vi "PH_Sequencer_Watch.PC _PUcharged.vi"(0 "i ref in":refnum<vi>, 2 "Tagname":string, 3 "Tagvalue":i32, 4 "no link":bool, 5 "error in (no error)":errorcluster) -> (14 "i ref out":refnum<vi>, 19 "error out":errorcluster)   [LabVIEW 2014, in "PH_Sequencer_Watch.lvlib"]
doc: "This VI writes the incoming information for measured voltage to the related GUI element and to own attributes."
uses:
  PH_Sequencer_Watch.lvlib
  PH_Basics/PH_PowerUnit_BaseClass/PH_PowerUnit_BaseClass.PP PU Tags.ctl
  PH_Basics/PH_PowerUnit_BaseClass/PH_PowerUnit_BaseClass.lvlib
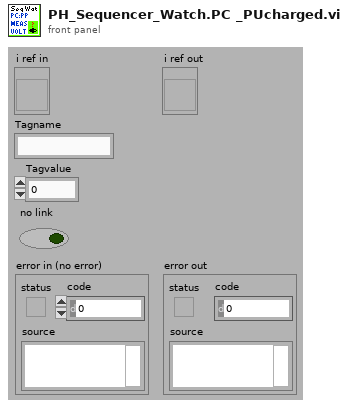
[diagram p1: front panel]
types:
  T1 = typedef "PH_Sequencer_Watch.lvlib/PH_Sequencer_Watch.i attribute.ctl" = cluster{"GUI Refs":cluster{"Shot ID":refnum<vi>, "Sequencer SM State":refnum<vi>, "Remaining Time":refnum<vi>, "PHELIX_Timing_T2":refnum<vi>, "T2-Unit-Dummy":refnum<vi>, "fs_Synchrolock_Watch":refnum<vi>, "Experiment_Vacuum_Control_Experiment":refnum<vi>}, "Status Synchrolock":T2, "Exp - Pressure":dbl, "Exp - Limit":dbl, "Heads":T3[], "Refs BooleanState":refnum<vi>[]}
  T2 = typedef "PH_StatusHandler.lvlib/PH_StatusHandler.Status.ctl" = i16
  T3 = typedef "PH_Sequencer_Watch.lvlib/PH_Sequencer_Watch.Head Information.ctl" = cluster{"Ref Volt":refnum<vi>, "PU":T4}
  T4 = typedef "PH_PP_Common.lvlib/PH_PP_Common.PUs.ctl" = enum16{"no Info", "PA-19mm-1", "PA-19mm-2", "PA-45mm-PILC", "PA-45mm-MAIN", "MA-PU-1", "MA-PU-2", "MA-PU-3", "MA-PU-4", "MA-PU-5", "MA-PU-6", "MA-FR", "MA-PILC", "PA-45mm-DP"}
  T5 = typedef "PH_PowerUnit_BaseClass.lvlib/PH_PowerUnit_BaseClass.PP PU Tags.ctl" = enum16{"Waiting-Time", "PU-in-Use"}
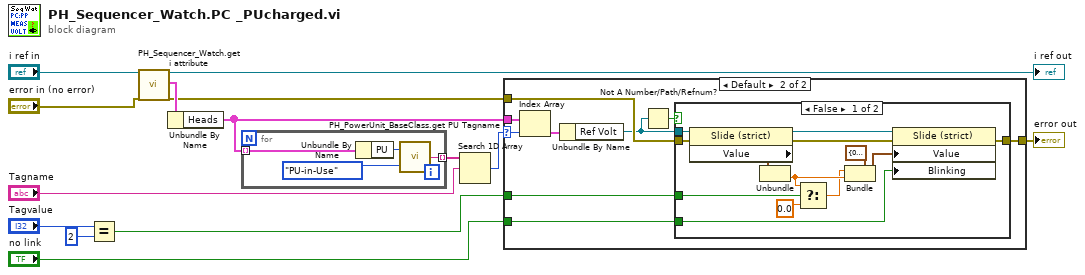
[diagram p0: block diagram]
diagram:
  n1 = Equal?(x="Tagvalue", y=2) -> (x = y?=w1:bool)
  n2 = call "PH_Sequencer_Watch.get i attribute.vi"("i ref in"="i ref in", "error in (no error)"="error in (no error)") -> ("i ref out"=→"i ref out":refnum<vi>, "i attribute"=w12:T1, "error out"=w8:errorcluster)  [unwired: 15 in]
  n3 = Unbundle By Name(w12) -> ("Heads"=w7:T3[])
  n4 = for {
    tunnel: w7 -> [w18] mode=indexing
    tunnel: [w16] -> w6 mode=indexing
    n5 = Unbundle By Name(w18) -> ("PU"=w17:T4)
    n6 = call "PH_PowerUnit_BaseClass.get PU Tagname.vi"("PU Tag"=PH_PowerUnit_BaseClass.PP_PU_Tags."PU-in-Use", "PU"=w17) -> ("PU Tagname"=w16:string)
  }
  n7 = Search 1D Array(1D array=w6, element="Tagname") -> (index of element=w4:i32)  [unwired: 1 in]
  n8 = case shown="Default" w4 {
    selector: w4 -> [_ w20]
    tunnel: [w19 w28] -> w11
    tunnel: w1 -> [_ w27]
    tunnel: "no link" -> [_ w26]
    tunnel: w8 -> [w19 w25]
    tunnel: w7 -> [_ w24]
    frame -1 {
    }
    frame Default {
      n9 = Index Array(array=w24, index=w20) -> (element=w22:T3)
      n10 = Unbundle By Name(w22) -> ("Ref Volt"=w21:refnum<vi>)
      n11 = Not A Number/Path/Refnum?(number/path/refnum=w21) -> (NaN/Path/Refnum?=w23:bool)
      n12 = case shown="False" w23 {
        tunnel: w21 -> [w36 _]
        tunnel: w25 -> [w40 w42]
        tunnel: [w39 w42] -> w28
        tunnel: w27 -> [w32 _]
        tunnel: w26 -> [w37 _]
        frame False {
          n13 = property class="Slide (strict)"(reference=w36, error in=w40) -> (reference out=w38:refnum<vi>, error out=w41:errorcluster, "Value"=w35:cluster{dbl, dbl})
          n14 = Unbundle(w35) -> (w31:dbl)  [unwired: 1 out]
          n15 = Select(t=w31, s=w32, f=0.0) -> (s? t:f=w30:dbl)
          n16 = Bundle(cluster=cluster{dbl, dbl} {0.0, 0.0} ("Value"), w30, w31) -> (w34:cluster{dbl, dbl})
          n17 = property class="Slide (strict)"(reference=w38, error in=w41, "Value"=w34, "Blinking"=w37) -> (error out=w39:errorcluster)  [unwired: 1 out]
        }
        frame True {
        }
      }
    }
  }
  "error out" <- w11
